vi "main_5.vi"(0 "Num 1":dbl=1.0 format="%#_13g", 5 "Num 2":dbl=3.0 format="%#_13g", 7 "Operation":T1, 11 "error in (no error)":errorcluster) -> (4 "return value":dbl, 15 "error out":errorcluster)   [LabVIEW 2023, in "task_5.lvlib"]
doc: "Do the math operations by calling a python script"
uses:
  task_5.lvlib
  Controls/operation_selector.ctl
panel:
  in  "Stop":bool
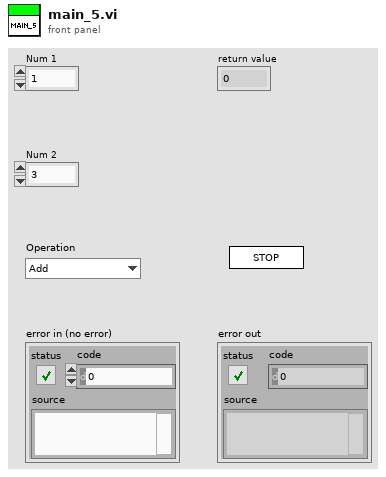
[diagram p1: front panel]
types:
  T1 = typedef "operation_selector.ctl" = enum16{"Add", "Subtract", "Divide", "Multiply"}
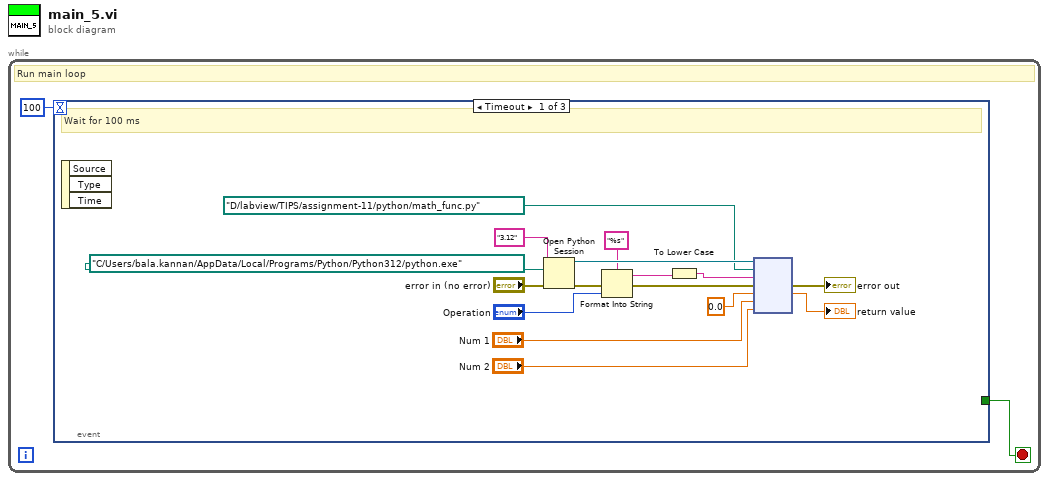
[diagram p0: block diagram]
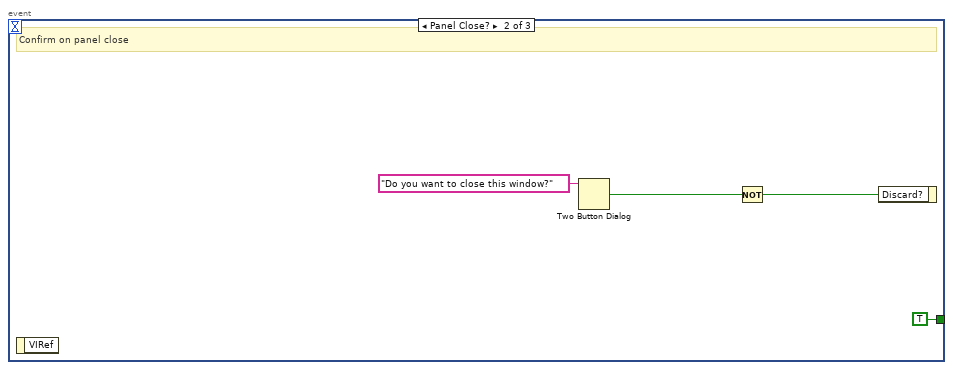
[diagram p2: hidden frame]
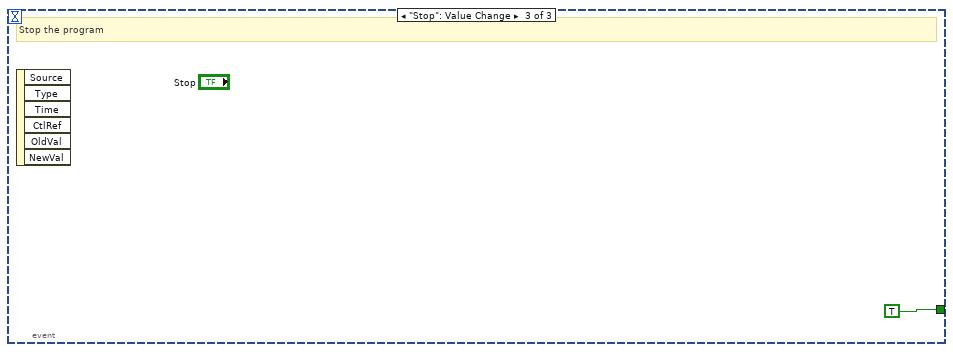
[diagram p3: hidden frame]
diagram:
  n1 = while {
    stop <- w1 stop-if-true
    # "Run main loop"
    n2 = event shown="[0] Timeout" {
      selector: _ -> [_ _ _]
      dyn-events: _ -> [_ _ _]
      timeout: 100 -> [_ _ _]
      tunnel: [_ TRUE TRUE] -> w1
      event Timeout {
        # "Wait for 100 ms"
        n3 = event-data() -> ()  [unwired: 1 in, 3 out]
        n4 = Open Python Session(python version="3.12" ("Python version"), python path=path "C:/Users/bala.kannan/AppData/Local/Programs/Python/Python312/python.exe" ("Python path"), 3:"error in (no error)") -> (session out=w18:refnum<k35>, error out=w7:errorcluster)
        n5 = Format Into String(format string="%s", error in=w7, "Operation") -> (resulting string=w4:string, error out=w6:errorcluster)  [unwired: 1 in]
        n6 = To Lower Case(string=w4) -> (all lower case string=w5:string)
        n7 = node(w18, path "D:/labview/TIPS/assignment-11/python/math_func.py" ("module path"), w5, w6, 0.0, "Num 1", "Num 2") -> (→"error out":errorcluster, →"return value":dbl)  [unwired: 2 in, 3 out]
      }
      event Panel Close? {
        # "Confirm on panel close"
        n8 = event-data() -> ()  [unwired: 1 in, 1 out]
        n9 = Two Button Dialog(message="Do you want to close this window?") -> (T button?=w21:bool)  [unwired: 2 in]
        n10 = Not(x=w21) -> (.not. x?=w20:bool)
        n11 = event-data("Discard?"=w20) -> ()  [unwired: 1 in, 1 out]
      }
      event "Stop": Value Change {
        # "Stop the program"
        n12 = event-data() -> ()  [unwired: 1 in, 6 out]
      }
    }
  }
